vi "Main.vi"() -> ()   [LabVIEW 2021]
panel:
  in  "Directory":path
  out "Image Out":T1(plugin-control)
  out "IR Flag":bool
  in  "Take Photo Button":bool
  out "Stop Flag":bool
  in  "Matching Button":bool
  in  "Open Button":bool
  in  "Create Pattern Button":bool
  in  "Stop Button":bool caption="Stop"
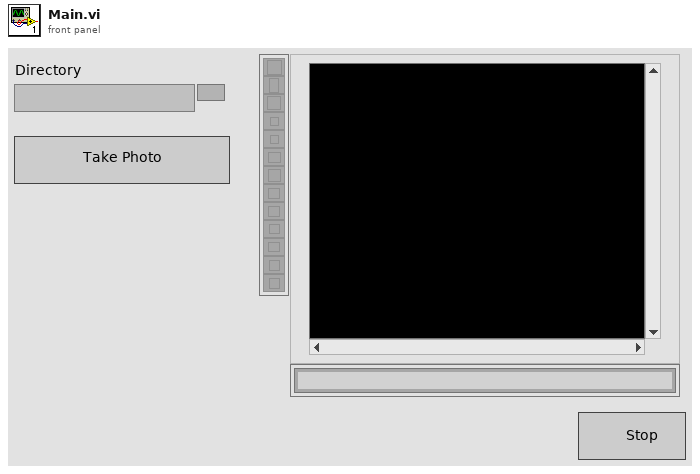
[diagram p1: front panel]
types:
  T1 = typedef "IMAQ Image.ctl" = refnum<image>
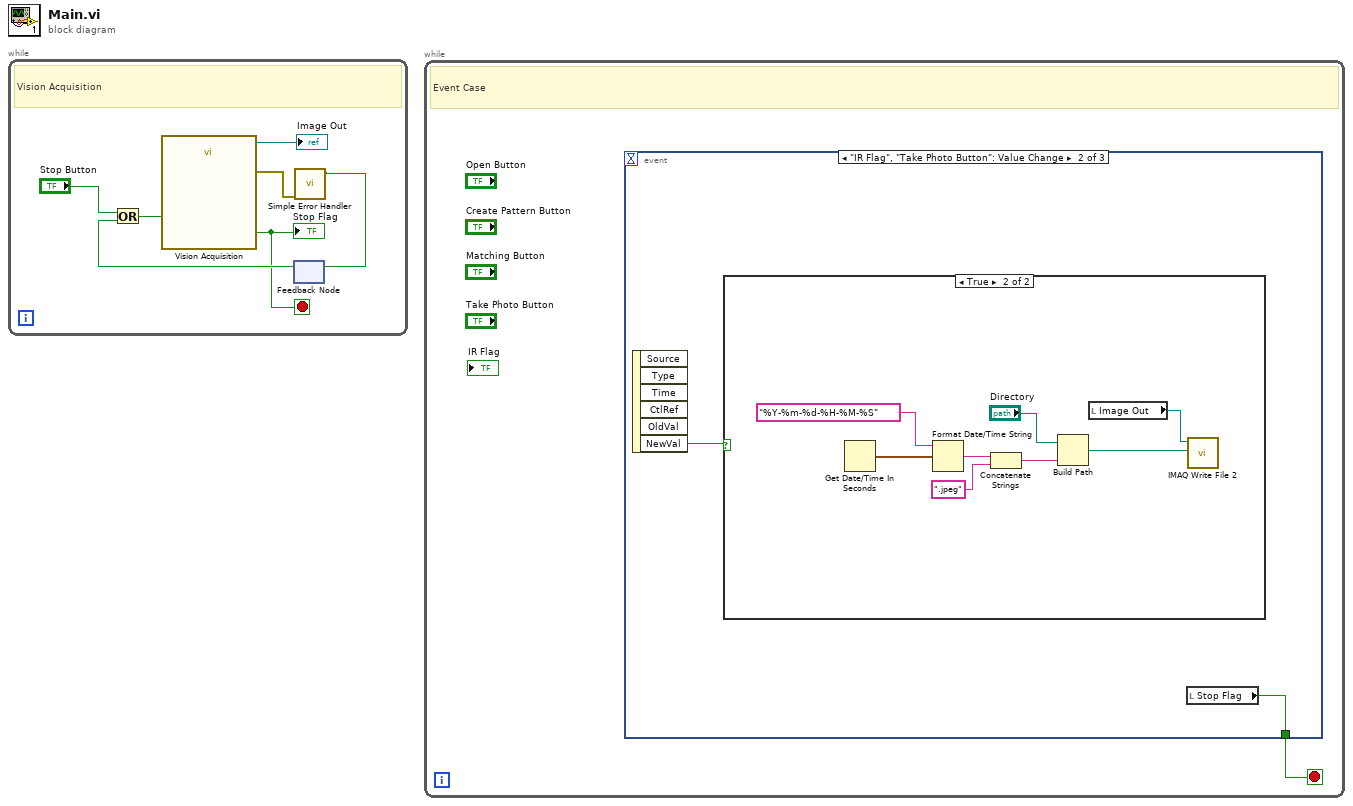
[diagram p0: block diagram]
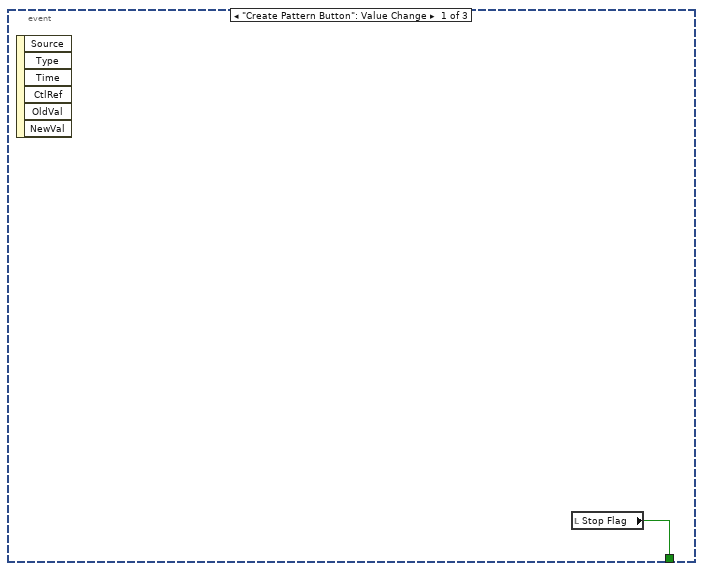
[diagram p2: hidden frame]
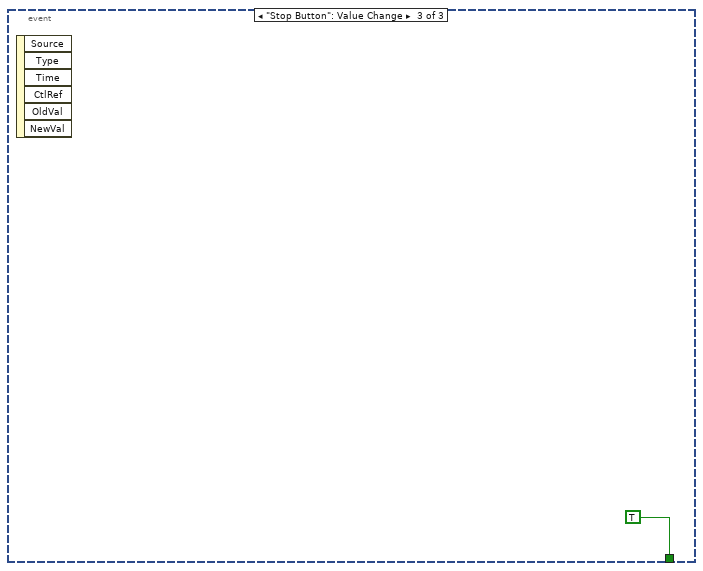
[diagram p4: hidden frame]
diagram:
  n1 = while {
    stop <- w2 stop-if-true
    # "Vision Acquisition"
    n2 = feedback #1() -> (w3:bool)  [unwired: 1 in]
    n3 = Or(x="Stop Button", y=w3) -> (x .or. y?=w6:bool)
    n4 = call "Vision Acquisition"("Stop (F)"=w6) -> ("Image Out"=→"Image Out":T1, "Stopped"=w2:bool, "error out"=w7:errorcluster)  [unwired: 24 in]
    "Stop Flag" <- w2
    n5 = call <vilib>:"Simple Error Handler.vi"("error in (no error)"=w7) -> ("error?"=w4:bool)  [unwired: 4 in, 4 out]
    n6 = feedback-in #1(w4) -> ()
  }
  n7 = while {
    stop <- w8 stop-if-true
    # "Event Case"
    n8 = event shown="[1] \"IR Flag\", \"Take Photo Button\": Value Change" {
      selector: _ -> [_ _ _]
      dyn-events: _ -> [_ _ _]
      timeout: _ -> [_ _ _]
      tunnel: [w9 w10 TRUE] -> w8
      event "Create Pattern Button": Value Change {
        n9 = event-data() -> ()  [unwired: 1 in, 6 out]
        n10 = local read "Stop Flag"() -> (w9:bool)
      }
      event "IR Flag", "Take Photo Button": Value Change {
        n11 = event-data() -> ("NewVal"=w11:bool)  [unwired: 1 in, 5 out]
        n12 = case shown="True" w11 {
          frame False {
          }
          frame True {
            n13 = Get Date/Time In Seconds() -> (seconds since 1Jan1904=w17:timestamp)
            n14 = Format Date/Time String(time format string (%c)="%Y-%m-%d-%H-%M-%S", seconds (now)=w17) -> (date/time string=w18:string)  [unwired: 1 in]
            n15 = Concatenate Strings(w18, ".jpeg" ("string")) -> (w12:string)
            n16 = Build Path(base path="Directory", name or relative path=w12) -> (appended path=w13:path)
            n17 = local read "Image Out"() -> (w19:T1)
            n18 = call-poly "IMAQ Write File 2"("File Path"=w13, "Image"=w19) -> ()  [unwired: 8 in, 2 out]
          }
        }
        n19 = local read "Stop Flag"() -> (w10:bool)
      }
      event "Stop Button": Value Change {
        n20 = event-data() -> ()  [unwired: 1 in, 6 out]
      }
    }
  }
